vi "_PC_DataChrom_Conv_GraphData.vi"(6 "Data State":enum16{"Mass", "XIC"}(ring), 7 "FilePath":path, 9 "Information":string[](array[string]), 11 "DataArray":cluster{"X":dbl[], "Y":dbl[]}[](array[cluster])) -> (3 "Output":T1)   [LabVIEW 2018]
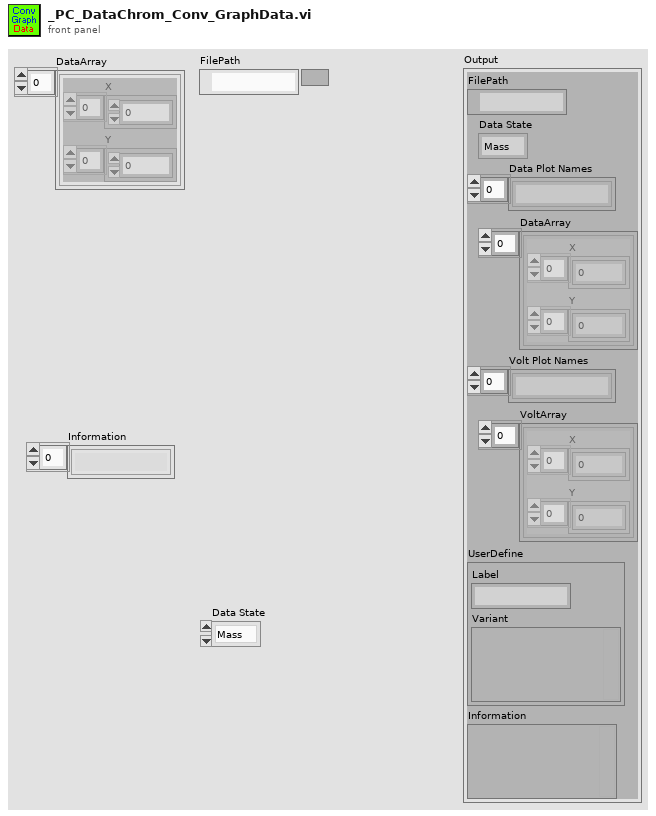
[diagram p1: front panel]
types:
  T1 = cluster{"FilePath":path, "Data State":enum16{"Mass", "XIC"}, "Data Plot Names":string[], "DataArray":cluster{"X":dbl[], "Y":dbl[]}[], "Volt Plot Names":string[], "VoltArray":cluster{"X":dbl[], "Y":dbl[]}[], "UserDefine":cluster{"Label":string, "Variant":variant}, "Information":variant}
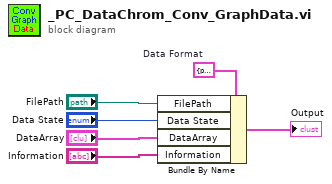
[diagram p0: block diagram]
diagram:
  w3 = T1 {"FilePath"=path "", "Data State"=enum."Mass", "Data Plot Names"=[], "DataArray"=[], "Volt Plot Names"=[], "VoltArray"=[], "UserDefine"={"Label"="", "Variant"=variant}, "Information"=variant}  # Data Format
  n1 = Bundle By Name(cluster=w3, "FilePath"="FilePath", "Data State"="Data State", "DataArray"="DataArray", "Information"="Information") -> (→"Output":T1)
